vi "Buffer Initialize.vi"(8 "error in (no error)":errorcluster, 9 "Number Of Elements":i32[](array[numeric]), 10 "Sector Number":i32, 11 "2D U16 DVR Array in":refnum<class "2D U16 DVR Array.lvclass">) -> (0 "error out":errorcluster, 3 "2D U16 DVR Array out":refnum<class "2D U16 DVR Array.lvclass">)   [LabVIEW 2024, in "2D U16 DVR Array.lvclass"]
uses:
  2D U16 DVR Array.lvclass
  2D U16 DVR Array.lvclass/2D U16 DVR Array.ctl
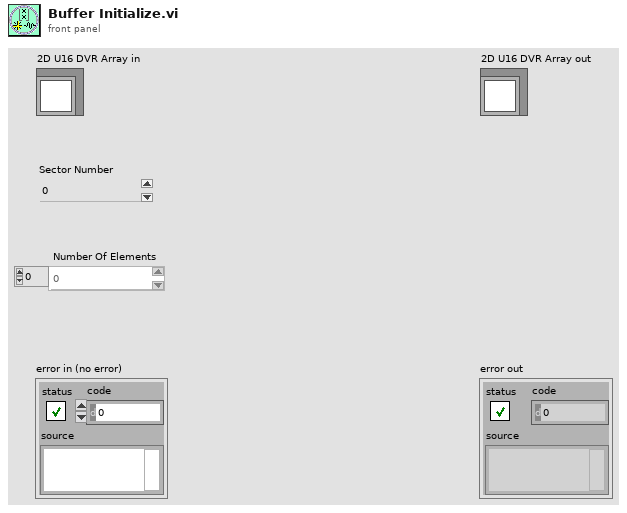
[diagram p1: front panel]
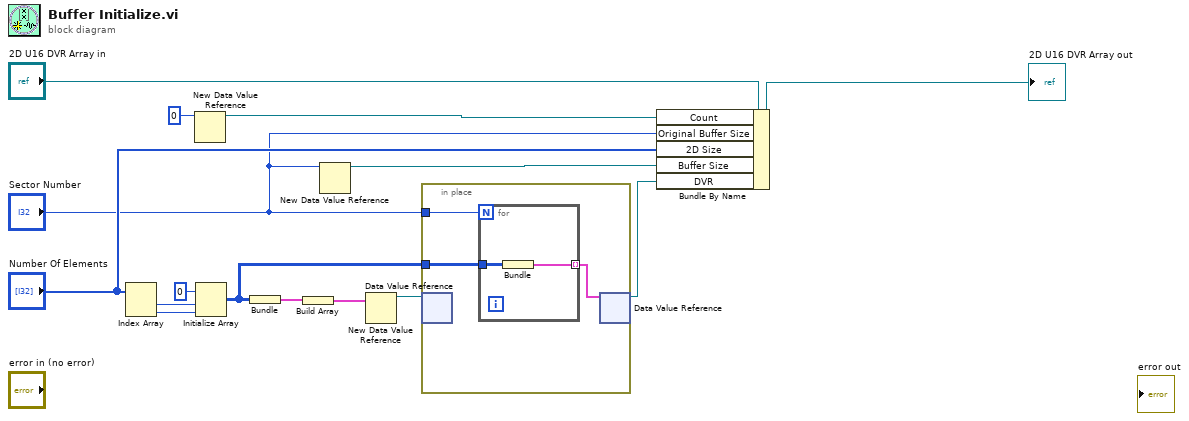
[diagram p0: block diagram]
diagram:
  n1 = Index Array(array="Number Of Elements") -> (element #1=w12:i32, element #2=w11:i32)  [unwired: 2 in]
  n2 = New Data Value Reference(data value=0 ("Sector Number")) -> (data value reference=w2:refnum<data-value>)  [unwired: 1 in, 1 out]
  n3 = Initialize Array(u16 0 ("element"), w12, w11) -> (w7:u16[][])
  n4 = Bundle(w7) -> (w10:cluster{u16[][]})  [unwired: 1 in]
  n5 = Build Array(w10) -> (w9:cluster{u16[][]}[])
  n6 = New Data Value Reference(data value="Sector Number") -> (data value reference=w4:refnum<data-value>)  [unwired: 1 in, 1 out]
  n7 = New Data Value Reference(data value=w9) -> (data value reference=w8:refnum<data-value>)  [unwired: 1 in, 1 out]
  n8 = in-place {
    in-place-border: "Sector Number" -> [w18]
    in-place-border: w7 -> [w17]
    n9 = in-place-dvr #1(w8) -> ()  [unwired: 2 out]
    n10 = for {
      N: w18 -> [_]
      tunnel: w17 -> [w20]
      tunnel: [w19] -> w16 mode=indexing
      n11 = Bundle(w20) -> (w19:cluster{u16[][]})  [unwired: 1 in]
    }
    n12 = in-place-dvr #1(w16) -> (w6:refnum<data-value>)  [unwired: 1 out]
  }
  n13 = Bundle By Name(cluster="2D U16 DVR Array in", "Count"=w2, "Original Buffer Size"="Sector Number", "2D Size"="Number Of Elements", "Buffer Size"=w4, "DVR"=w6) -> (→"2D U16 DVR Array out":refnum<class "2D U16 DVR Array.lvclass">)
